vi "Stream ALL Velocity Values.vi"(6 "Output Values":dbl[](array[numeric]), 7 "Motor List":T1[](array[typedef]), 8 "Output Times":dbl[](array[numeric]), 9 "Drive Target Values":dbl[](array[numeric]), 10 "Drive Velocity Values":dbl[](array[numeric]), 11 "Drive Times":dbl[](array[numeric])) -> ()   [LabVIEW 2020, in "SwerveDrive_ACT.lvlib"]
uses:
  SwerveDrive_ACT.lvlib
  Shared Code/TypeDefs/ENUM_Motor Index.ctl
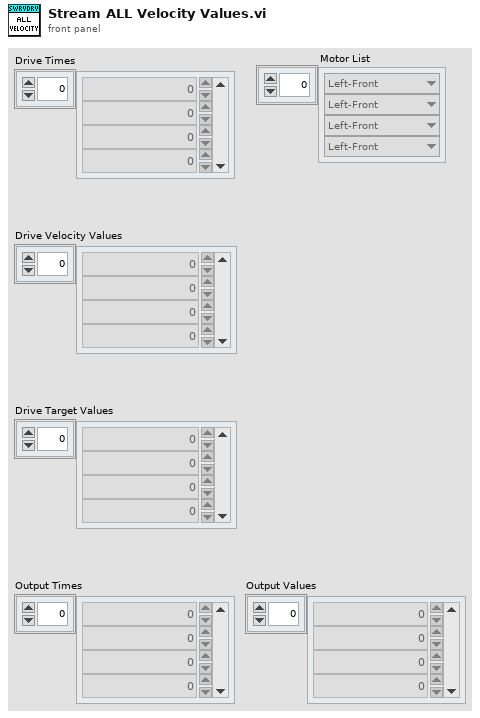
[diagram p1: front panel]
types:
  T1 = typedef "ENUM_Motor Index.ctl" = enum16{"Left-Front", "Right-Front", "Left-Back", "Right-Back"}
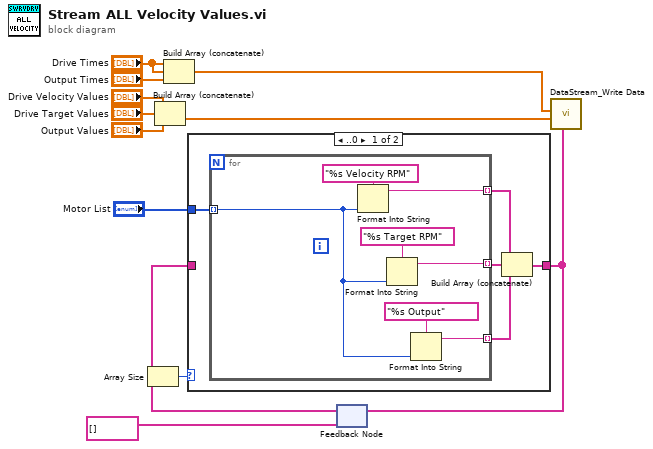
[diagram p0: block diagram]
diagram:
  n1 = Build Array (concatenate)("Drive Velocity Values", "Drive Target Values", "Output Values") -> (w2:dbl[])
  n2 = Build Array (concatenate)("Drive Times", "Drive Times", "Output Times") -> (w8:dbl[])
  n3 = feedback #1(string[] []) -> (w10:string[])
  n4 = Array Size(array=w10) -> (size(s)=w11:i32)
  n5 = case shown="..0" w11 {
    tunnel: w10 -> [_ w25]
    tunnel: [w13 w25] -> w9
    tunnel: "Motor List" -> [w17 _]
    frame ..0 {
      n6 = for {
        tunnel: w17 -> [w18] mode=indexing
        tunnel: [w23] -> w16 mode=indexing
        tunnel: [w21] -> w15 mode=indexing
        tunnel: [w19] -> w14 mode=indexing
        n7 = Format Into String(format string="%s Velocity RPM", w18) -> (resulting string=w23:string)  [unwired: 2 in, 1 out]
        n8 = Format Into String(format string="%s Target RPM", w18) -> (resulting string=w21:string)  [unwired: 2 in, 1 out]
        n9 = Format Into String(format string="%s Output", w18) -> (resulting string=w19:string)  [unwired: 2 in, 1 out]
      }
      n10 = Build Array (concatenate)(w16, w15, w14) -> (w13:string[])
    }
    frame 1.. {
    }
  }
  n11 = feedback-in #1(w9) -> ()
  n12 = call "DataStream_Write Data.vi"("Header Array"=w9, "Value Array"=w2, "Time Stamp Array"=w8) -> ()  [unwired: 7 in, 2 out]
